vi "Get Value from Database.vi"(8 "error in (no error)":errorcluster, 10 "Measurement Name":string, 11 "Multi Step Database in":refnum<class "Multi Step Database.lvclass">) -> (0 "error out":errorcluster, 2 "Measurement Definition":T1[](array[typedef]), 3 "Multi Step Database out":refnum<class "Multi Step Database.lvclass">)   [LabVIEW 2016, in "NI Generic Parser.lvlib" / "Multi Step Database.lvclass"]
uses:
  Multi Step Database.lvclass
  Plugins/Measurement Data.lvlibp/Controls/Measurement Description.ctl
  Plugins/String Database.lvlibp/String Database.lvclass
  Plugins/Measurement Data.lvlibp/Controls/Measurement Position.ctl
  Multi Step Database.lvclass/Multi Step Database.ctl
  <vilib>/Utility/error.llb/Error Cluster From Error Code.vi
  <vilib>/ErrorRing/Error Ring.xnode
  Plugins/Measurement Data.lvlibp/Measurement Data.lvclass
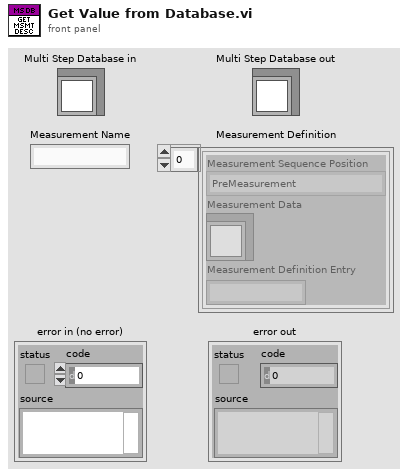
[diagram p1: front panel]
types:
  T1 = typedef "Measurement Data.lvlibp/Measurement Data.lvclass/Measurement Description.ctl" = cluster{"Measurement Sequence Position":T2, "Measurement Data":refnum<class "String Database.lvclass">, "Measurement Definition Entry":string}
  T2 = typedef "Measurement Data.lvlibp/Measurement Data.lvclass/Measurement Position.ctl" = enum16{"PreMeasurement", "MainMeasurement", "PostMeasurement"}
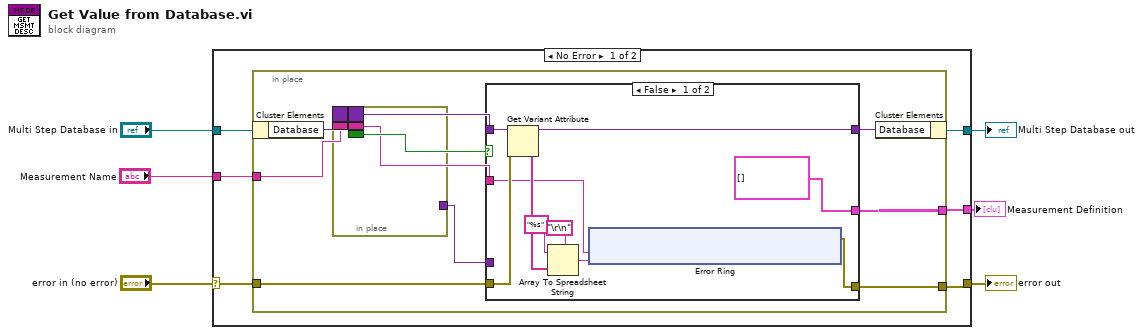
[diagram p0: block diagram]
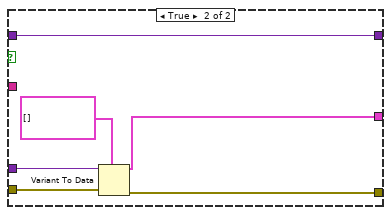
[diagram p2: hidden frame]
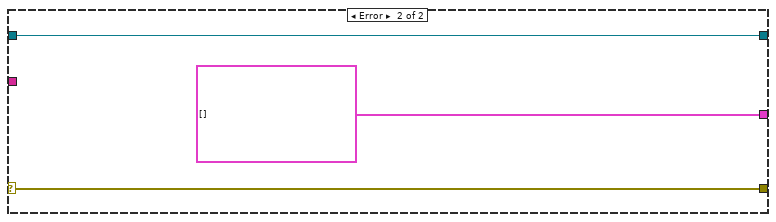
[diagram p3: hidden frame]
diagram:
  n1 = case shown="No Error" "error in (no error)" {
    selector: "error in (no error)" -> [w8 w50]
    tunnel: [w9 w50] -> w5
    tunnel: "Multi Step Database in" -> [w12 w49]
    tunnel: "Measurement Name" -> [w11 _]
    tunnel: [w10 w49] -> w2
    tunnel: [w7 T1[] [] ("Array")] -> w1
    frame No Error {
      n2 = in-place {
        in-place-border: w11 -> [w21]
        in-place-border: [w19] -> w9
        in-place-border: w8 -> [w18]
        in-place-border: [w17] -> w7
        n3 = in-place-cluster #1(w12) -> ("Database"=w22:variant)
        n4 = in-place {
          border: w22 -> [_]
          border: w21 -> [_]
          border: [_] -> w14
          border: [_] -> w13
          border: [_] -> w16
          in-place-border: [w23] -> w20
        }
        n5 = case shown="False" w16 {
          tunnel: w20 -> [_ w47]
          tunnel: [w28 w45] -> w19
          tunnel: w18 -> [w30 w44]
          tunnel: [T1[] [] ("Array") w43] -> w17
          tunnel: [w31 w42] -> w15
          tunnel: w14 -> [w33 w42]
          tunnel: w13 -> [w24 _]
          frame False {
            n6 = Get Variant Attribute(Variant=w33, error in=w30) -> (duplicate Variant=w31:variant, names=w29:string[])  [unwired: 2 in, 2 out]
            n7 = Array To Spreadsheet String(delimiter (Tab)="\r\n", array=w29, 3:"%s" ("format string")) -> (spreadsheet string=w26:string)
            n8 = xnode "Error Ring"("parameter 0"=w24, "parameter 1"=w26) -> ("error out"=w28:errorcluster)
          }
          frame True {
            n9 = Variant To Data(error in=w44, type=T1[] [] ("Array"), Variant=w47) -> (data=w43:T1[], error out=w45:errorcluster)
          }
        }
        n10 = in-place-cluster #1("Database"=w15) -> (w10:refnum<class "Multi Step Database.lvclass">)
      }
    }
    frame Error {
    }
  }
  "error out" <- w5
  "Multi Step Database out" <- w2
  "Measurement Definition" <- w1
